vi "Constructor.vi"(8 "error in (no error)":errorcluster) -> (0 "error out":errorcluster, 2 "Mouse":refnum<event-registration>, 3 "Mouse out":refnum<class "Mouse.lvclass">)   [LabVIEW 2021, in "InputDevice.lvlib" / "Mouse.lvclass"]
uses:
  Mouse.lvclass
  data.ctl
  Mouse.lvclass/Mouse.ctl
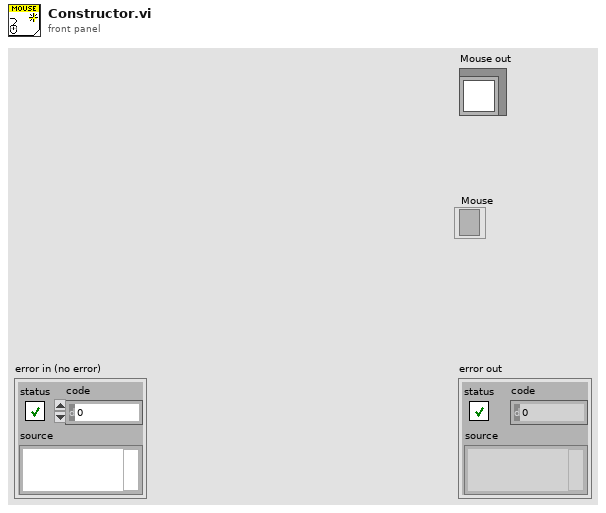
[diagram p1: front panel]
types:
  T1 = typedef "InputDevice.lvlib/Mouse.lvclass/data.ctl" = cluster{"DeviceID":refnum<k1>, "MouseButtonInfo":refnum<user-event>, "MouseAxisInfo":refnum<user-event>, "MouseInfoEvents":refnum<event-registration>, "StopNotifier":refnum<notifier>}
  T2 = cluster{"Horizontal":i32, "Vertical":i32, "Scrolling":i32}
  T3 = cluster{"Button 1":bool, "Button 2":bool, "Button 3":bool, "Button 4":bool}
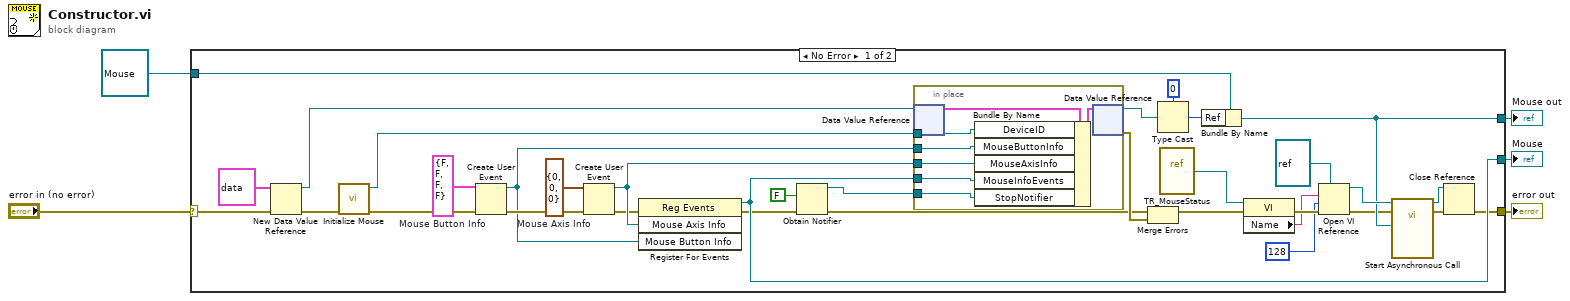
[diagram p0: block diagram]
diagram:
  n1 = case shown="No Error" "error in (no error)" {
    selector: "error in (no error)" -> [w33 w48]
    tunnel: [w7 w48] -> w4
    tunnel: [w11 w47] -> w3
    tunnel: refnum<class "Mouse.lvclass"> refnum ("Mouse.lvclass") -> [w37 w47]
    tunnel: [w22 _] -> w1
    frame No Error {
      w26 = T2 {"Horizontal"=0, "Vertical"=0, "Scrolling"=0}  # Mouse Axis Info
      w29 = T3 {"Button 1"=FALSE, "Button 2"=FALSE, "Button 3"=FALSE, "Button 4"=FALSE}  # Mouse Button Info
      n2 = New Data Value Reference(data value=T1 {"DeviceID"=refnum, "MouseButtonInfo"=refnum, "MouseAxisInfo"=refnum, "MouseInfoEvents"=refnum, "StopNotifier"=refnum} ("Cluster"), error in=w33) -> (data value reference=w38:refnum<data-value>, error out=w32:errorcluster)
      n3 = call <vilib>:"Initialize Mouse.vi"("error in (no error)"=w32) -> ("error out"=w28:errorcluster, "device ID"=w31:refnum<k1>)  [unwired: 9 in]
      n4 = Create User Event(user event datatype=w29, error in=w28) -> (user event=w24:refnum<user-event>, error out=w27:errorcluster)
      n5 = Create User Event(user event datatype=w26, error in=w27) -> (user event=w25:refnum<user-event>, error out=w23:errorcluster)
      n6 = register-events(error in=w23, w25, w24) -> (reference out=w22:refnum<event-registration>, error out=w20:errorcluster)  [unwired: 1 in]
      n7 = Obtain Notifier(notification data type=FALSE, error in (no error)=w20) -> (notifier out=w8:refnum<notifier>, error out=w19:errorcluster)  [unwired: 2 in, 1 out]
      n8 = in-place {
        in-place-border: w31 -> [w44]
        in-place-border: w24 -> [w43]
        in-place-border: w25 -> [w42]
        in-place-border: w22 -> [w41]
        in-place-border: w8 -> [w40]
        n9 = in-place-dvr #1(w38) -> (w46:T1)  [unwired: 1 out]
        n10 = Bundle By Name(cluster=w46, "DeviceID"=w44, "MouseButtonInfo"=w43, "MouseAxisInfo"=w42, "MouseInfoEvents"=w41, "StopNotifier"=w40) -> (w45:T1)
        n11 = in-place-dvr #1(w45) -> (w36:refnum<data-value>, w30:errorcluster)
      }
      n12 = Merge Errors(w19, w30) -> (w18:errorcluster)
      n13 = Type Cast(type=u64 0 ("Ref"), x=w36) -> (*(type *) &x=w34:u64)
      n14 = vi-ref "TR_MouseStatus.vi"() -> (w14:refnum<vi>)
      n15 = Bundle By Name(cluster=w37, "Ref"=w34) -> (w11:refnum<class "Mouse.lvclass">)
      n16 = property class="VI"(reference=w14, error in=w18) -> (error out=w17:errorcluster, "Name"=w16:string)  [unwired: 1 out]
      n17 = Open VI Reference(type specifier VI Refnum (for type only)=refnum<vi> refnum, vi path=w16, options=128, error in (no error)=w17) -> (vi reference=w13:refnum<vi>, error out=w10:errorcluster)  [unwired: 2 in]
      n18 = call-by-ref "Start Asynchronous Call"(reference=w13, error in=w10, "Mouse in"=w11) -> (reference out=w6:refnum<vi>, error out=w9:errorcluster)  [unwired: 11 in]
      n19 = Close Reference(reference=w6, error in (no error)=w9) -> (error out=w7:errorcluster)
    }
    frame Error {
    }
  }
  "error out" <- w4
  "Mouse out" <- w3
  "Mouse" <- w1
